vi "Malleable VIs Basics Lesson 1.vi"() -> ()   [LabVIEW 2023]
doc: "Introduction to the malleable VIs feature."
uses:
  <vilib>/Array/Sort 2D Array - Pop Stack.vi
  <vilib>/Array/Sort 2D Array - Push Stack.vi
panel:
  out "String":string
  out "Value Changed":bool[](array[boolean])
  out "Array with Incremented Element":i32[](array[numeric])
  out "Shuffled 1D Array":i32[](array[numeric])
  out "Sorted 2D Array":string[][](array[string])
  # "Overview: Introduction to the malleable VIs feature. Malleable VIs are so named because they mold themselves to fit their callers.\n\nInstructions: \n1. Open the block diagram of this VI. Review the lessons presented there.\n2. Run the VI to see the outputs displayed on the panel.\n3. Once you have finished reviewing this VI, open the Lesson 2 VI in the Malleable VIs Basics example project."
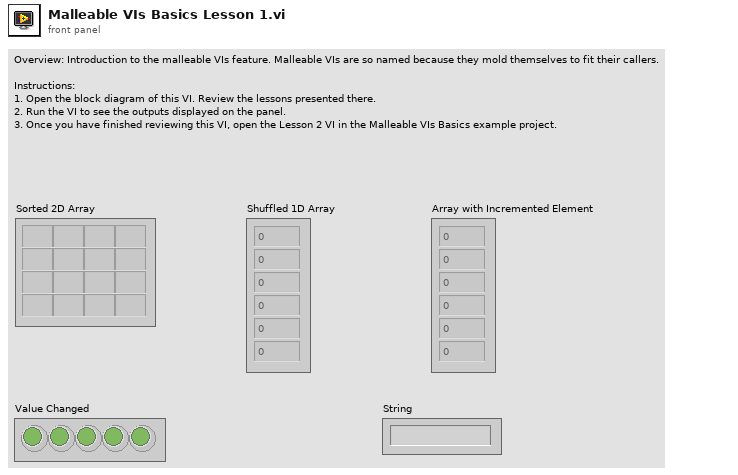
[diagram p1: front panel]
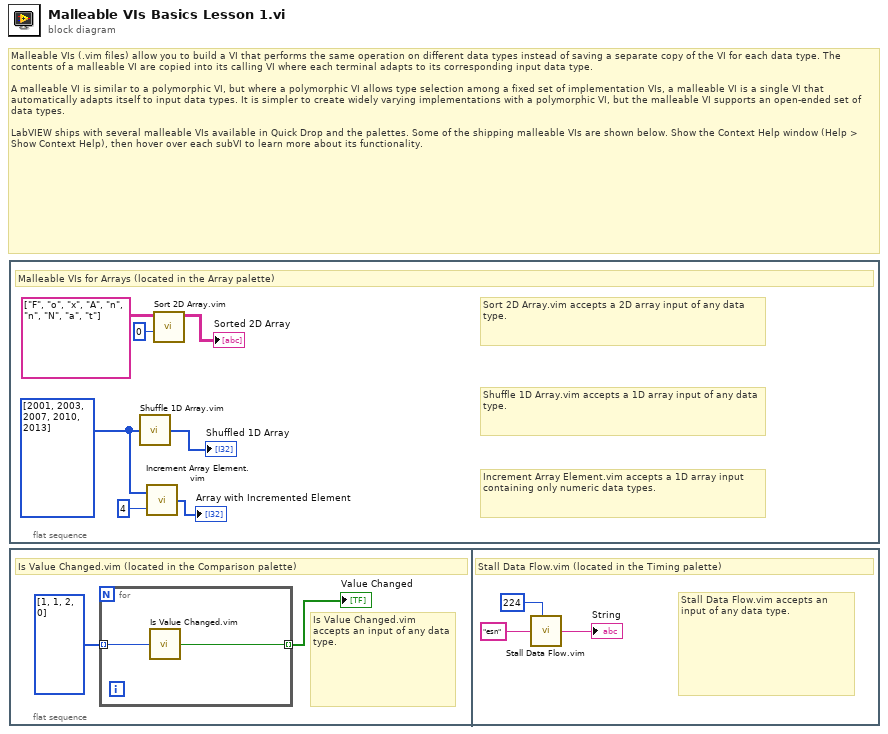
[diagram p0: block diagram]
diagram:
  # "Malleable VIs (.vim files) allow you to build a VI that performs the same operation on different data types instead of saving a separate copy of the VI for each data type. The contents of a malleable VI are copied into its calling VI where each terminal adapts to its corresponding input data type.\n\nA malleable VI is similar to a polymorphic VI, but where a polymorphic VI allows type selection among a fixed set of implementation VIs, a malleable VI is a single VI that automatically adapts itself to input data types. It is simpler to create widely varying implementations with a polymorphic VI, but the malleable VI supports an open-ended set of data types.\n\nLabVIEW ships with several malleable VIs available in Quick Drop and the palettes. Some of the shipping malleable VIs are shown below. Show the Context Help window (Help > Show Context Help), then hover over each subVI to learn more about its functionality."
  n1 = flat-sequence {
    frame #0 {
      w3 = i32[] [2001, 2003, 2007, 2010, 2013]
      # "Increment Array Element.vim accepts a 1D array input containing only numeric data types."
      # "Shuffle 1D Array.vim accepts a 1D array input of any data type."
      # "Sort 2D Array.vim accepts a 2D array input of any data type."
      # "Malleable VIs for Arrays (located in the Array palette)"
      n2 = call "Shuffle 1D Array.vim"("array"=w3) -> ("shuffled array"=→"Shuffled 1D Array":i32[])  [unwired: 4 in]
      n3 = call "Increment Array Element.vim"("index"=4, "array in"=w3) -> ("array out"=→"Array with Incremented Element":i32[])
      n4 = call "Sort 2D Array.vim"("index"=0, "2D array"=string[][] [["F", "o", "x"], ["A", "n", "n"], ["N", "a", "t"]]) -> ("sorted 2D array"=→"Sorted 2D Array":string[][])  [unwired: 8 in, 1 out]
    }
  }
  n5 = flat-sequence {
    frame #0 {
      # "Is Value Changed.vim accepts an input of any data type."
      # "Is Value Changed.vim (located in the Comparison palette)"
      n6 = for {
        tunnel: [w11] -> w9 mode=indexing
        tunnel: i32[] [1, 1, 2, 0] -> [w10] mode=indexing
        n7 = call "Is Value Changed.vim"("value"=w10) -> ("changed or first call?"=w11:bool)
      }
      "Value Changed" <- w9
    }
    frame #1 {
      # "Stall Data Flow.vim accepts an input of any data type."
      # "Stall Data Flow.vim (located in the Timing palette)"
      n8 = call "Stall Data Flow.vim"("value in"="esn", "milliseconds to wait"=u32 224) -> ("value out"=→"String":string)  [unwired: 1 out]
    }
  }
